vi "Test_CellOCV.vi"(7 "Limits":T2, 8 "error in (no error) 2":errorcluster, 11 "connection ID 2":refnum<k5>) -> (0 "error out 2":errorcluster, 1 "cell sum":dbl, 2 "delta V":dbl, 3 "connection ID out 2":refnum<k5>, 4 "worst cell V":dbl, 5 "results":T1(array[cluster]), 6 "worst cell":i32, 10 "cell volts":dbl[](array[numeric]))   [LabVIEW 2026]
uses:
  Limits.ctl
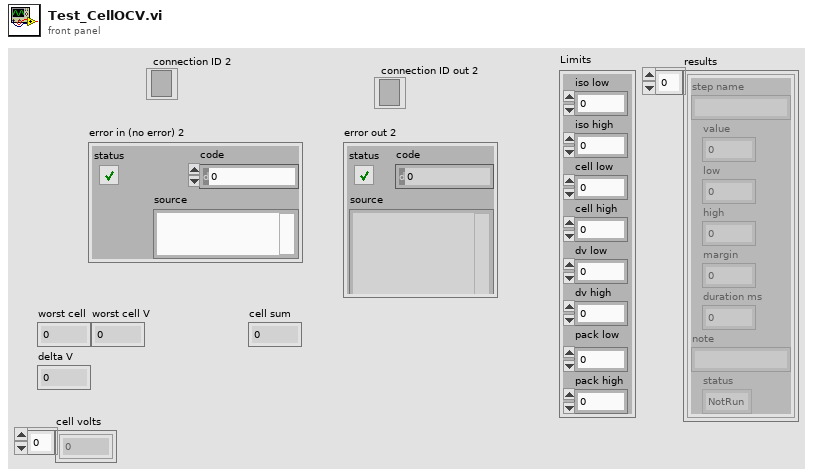
[diagram p1: front panel]
types:
  T1 = cluster{"step name":string, "value":dbl, "low":dbl, "high ":dbl, "margin":dbl, "duration ms":dbl, "note":string, "status":enum16{"NotRun", "Pass", "Fail", "Skipped"}}[]
  T2 = typedef "Limits.ctl" = cluster{"iso low":dbl, "iso high":dbl, "cell low":dbl, "cell high":dbl, "dv low":dbl, "dv high":dbl, "pack low":dbl, "pack high":dbl}
  T3 = cluster{"step name":string, "value":dbl, "low":dbl, "high ":dbl, "margin":dbl, "duration ms":dbl, "note":string, "status":enum16{"NotRun", "Pass", "Fail", "Skipped"}}
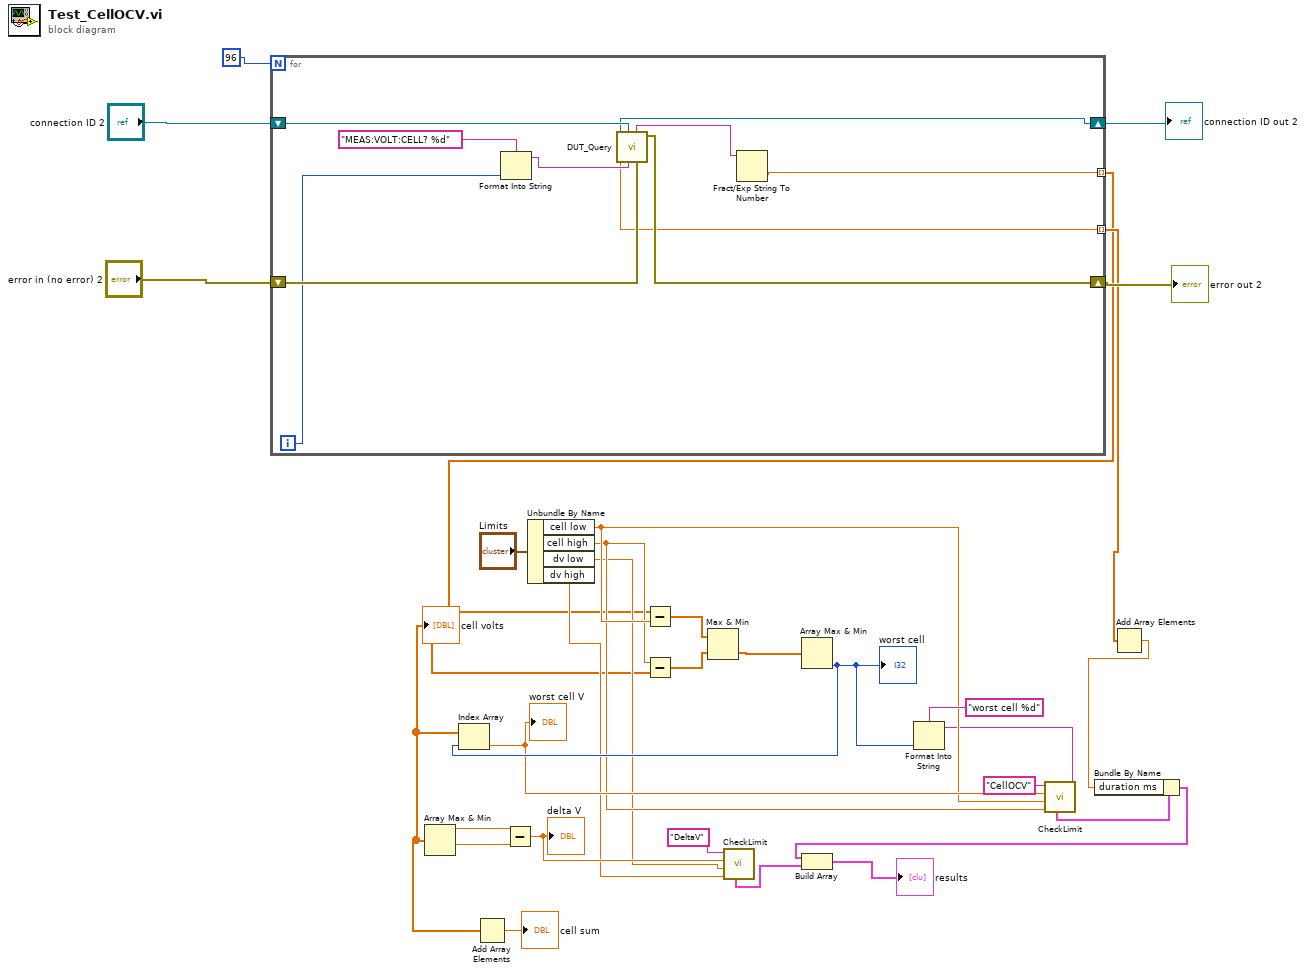
[diagram p0: block diagram]
diagram:
  n1 = for {
    N: 96 -> [_]
    shift-right: [w39] -> w27
    shift-left: "connection ID 2" -> [w40]
    shift-right: [w37] -> w26
    shift-left: "error in (no error) 2" -> [w38]
    tunnel: [w32] -> w2 mode=indexing
    tunnel: [w31] -> w25 mode=indexing
    i -> [w36]
    n2 = Format Into String(format string="MEAS:VOLT:CELL? %d", w36) -> (resulting string=w35:string)  [unwired: 2 in, 1 out]
    n3 = call "DUT_Query.vi"("error in (no error)"=w38, "command"=w35, "connection ID"=w40) -> ("error out"=w37:errorcluster, "reply"=w33:string, "elapsed ms"=w31:dbl, "connection ID out"=w39:refnum<k5>)  [unwired: 5 in]
    n4 = Fract/Exp String To Number(string=w33) -> (number=w32:dbl)  [unwired: 3 in, 1 out]
  }
  "connection ID out 2" <- w27
  "error out 2" <- w26
  "cell volts" <- w2
  n5 = Array Max & Min(array=w2) -> (max value=w11:dbl, min value=w10:dbl)  [unwired: 2 out]
  n6 = Add Array Elements(numeric array=w2) -> (sum=→"cell sum":dbl)
  n7 = Subtract(x=w11, y=w10) -> (x-y=w9:dbl)
  "delta V" <- w9
  n8 = Unbundle By Name("Limits") -> ("cell low"=w17:dbl, "cell high"=w16:dbl, "dv low"=w8:dbl, "dv high"=w7:dbl)
  n9 = Subtract(x=w2, y=w17) -> (x-y=w23:dbl[])
  n10 = Subtract(x=w16, y=w2) -> (x-y=w22:dbl[])
  n11 = Max & Min(x=w23, y=w22) -> (min(x,y)=w21:dbl[])  [unwired: 1 out]
  n12 = call "CheckLimit.vi"("high"=w7, "low"=w8, "value"=w9, "step name"="DeltaV") -> ("Result"=w4:T3)  [unwired: 5 in, 2 out]
  n13 = Array Max & Min(array=w21) -> (min index (indices)=w19:i32)  [unwired: 3 out]
  "worst cell" <- w19
  n14 = Index Array(array=w2, index=w19) -> (element=w18:dbl)
  "worst cell V" <- w18
  n15 = Format Into String(format string="worst cell %d", w19) -> (resulting string=w14:string)  [unwired: 2 in, 1 out]
  n16 = call "CheckLimit.vi"("note"=w14, "high"=w16, "low"=w17, "value"=w18, "step name"="CellOCV") -> ("Result"=w13:T3)  [unwired: 4 in, 2 out]
  n17 = Add Array Elements(numeric array=w25) -> (sum=w12:dbl)
  n18 = Bundle By Name(cluster=w13, "duration ms"=w12) -> (w5:T3)
  n19 = Build Array(w5, w4) -> (→"results":T1)
